vi "Send Exit.vi"(8 "ErrorIn":errorcluster, 11 "VISAIn":refnum<visa-resource-name>) -> (0 "ErrorOut":errorcluster, 2 "Data":string, 3 "VISAOut":refnum<visa-resource-name>)   [LabVIEW 2017, in "I28Drivers.lvlib"]
uses:
  I28Drivers.lvlib
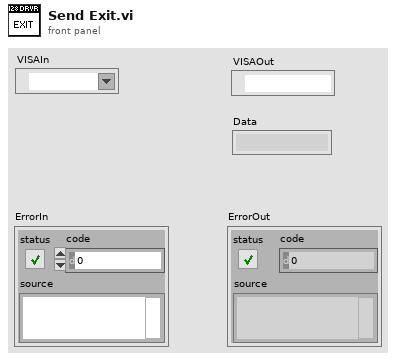
[diagram p1: front panel]
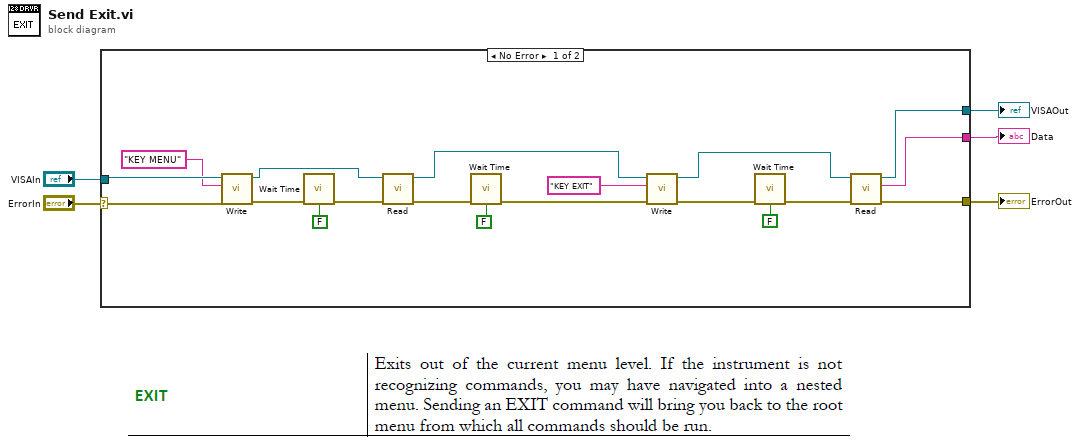
[diagram p0: block diagram]
diagram:
  n1 = case shown="No Error" "ErrorIn" {
    selector: "ErrorIn" -> [w20 w25]
    tunnel: "VISAIn" -> [w19 w26]
    tunnel: [w23 _] -> w3
    tunnel: [w22 w26] -> w1
    tunnel: [w21 w25] -> w2
    frame No Error {
      n2 = call "Write.vi"("ErrorIn"=w20, "Command"="KEY MENU", "VISAIn"=w19) -> ("ErrorOut"=w17:errorcluster, "VISAOut"=w15:refnum<visa-resource-name>)  [unwired: 7 in]
      n3 = call "Wait Time.vi"("error in"=w17, "Set Time"=FALSE) -> ("error out"=w16:errorcluster)  [unwired: 13 in]
      n4 = call "Read.vi"("ErrorIn"=w16, "VISAIn"=w15) -> ("ErrorOut"=w12:errorcluster, "VISAOut"=w13:refnum<visa-resource-name>)  [unwired: 7 in, 1 out]
      n5 = call "Wait Time.vi"("error in"=w12, "Set Time"=FALSE) -> ("error out"=w11:errorcluster)  [unwired: 13 in]
      n6 = call "Write.vi"("ErrorIn"=w11, "Command"="KEY EXIT", "VISAIn"=w13) -> ("ErrorOut"=w8:errorcluster, "VISAOut"=w9:refnum<visa-resource-name>)  [unwired: 7 in]
      n7 = call "Wait Time.vi"("error in"=w8, "Set Time"=FALSE) -> ("error out"=w7:errorcluster)  [unwired: 13 in]
      n8 = call "Read.vi"("ErrorIn"=w7, "VISAIn"=w9) -> ("ErrorOut"=w21:errorcluster, "Data"=w23:string, "VISAOut"=w22:refnum<visa-resource-name>)  [unwired: 7 in]
    }
    frame Error {
    }
  }
  "ErrorOut" <- w2
  "Data" <- w3
  "VISAOut" <- w1
